vi "Process.vi"(8 "error in":errorcluster, 11 "Inst.Transport in":refnum<class "Inst.Transport.lvclass">) -> (0 "error out":errorcluster, 3 "Inst.Transport out":refnum<class "Inst.Transport.lvclass">)   [LabVIEW 2019, in "Inst.Transport.lvclass"]
doc: "---------------------------------------------------------------\nJKI State Machine Objects™\nhttp://jki.net/state-machine-objects/\nCopyright (C) 2005-2015, JKI <info@jki.net>\nALL RIGHTS RESERVED"
uses:
  Inst.Transport.lvclass
  C:/Program Files (x86)/National Instruments/LabVIEW 2019/vi.lib/JKI/JKI SMO/SMO/SMO.lvclass
  C:/Program Files (x86)/National Instruments/LabVIEW 2019/user.lib/LevyLab/Instrument Framework/Instrument/Instrument.lvclass
  Typedefs/Inst.Transport.PublicCommands--Enum.ctl
  Typedefs/Inst.Transport.ProtectedCommands--Enum.ctl
  Typedefs/startTransport--Request--Cluster.ctl
  Typedefs/Inst.Transport.Methods--Enum.ctl
  Typedefs/setExptFolder--Request--Cluster.ctl
  Typedefs/setExptComments--Request--Cluster.ctl
  Typedefs/PrivateEvents--MessageToProcess.ctl
  <userlib>/LevyLab/RemoteControl/RemoteControl/Typedefs/Message--Cluster.ctl
  Inst.Transport.lvclass/Inst.Transport.ctl
  Transport/Transport.lvclass/Transport.ctl
  Typedefs/Inst.Transport.Status--Enum.ctl
  <vilib>/JKI/JKI SMO/SMO/SMO.lvclass/SMO.ctl
  Control Experiment/Control Experiment.lvclass
  Control Experiment/Control Experiment.lvclass/Control Experiment.ctl
  Transport/Typedefs/Lockin_Sweep JSON--Cluster.ctl
  <userlib>/LevyLab/Lockin-Multichannel/Instrument.DAQ/Typedefs/Sweep.Channel--Cluster--Array.ctl
  <userlib>/LevyLab/Lockin-Multichannel/Instrument.DAQ/Typedefs/Sweep.Channel--Cluster.ctl
  <userlib>/LevyLab/Lockin-Multichannel/Instrument.DAQ/Typedefs/Sweep.Pattern--Enum.ctl
  Typedefs/setSweepConfig--Request--Cluster.ctl
  41101f9e-a4cc-4be1-b6e3-cc7aeb9eb354.vi
  d30b621e-3614-4fe5-8996-767b375fe1bd.vi
  744a5e80-96fd-41c3-bea5-87d1f33fb3b4.vi
  079e2b50-2307-4fef-96c7-ae8985376933.vi
  0da1cde2-b360-4fd3-820f-4bad75bb71e2.vi
  853791a9-a17a-427f-8d0f-8733465fb5f1.vi
  744a5e80-96fd-41c3-bea5-87d1f33fb3b4.vi/ff32358f-5752-4f64-93da-f1ac2c9d74ec.vi
  744a5e80-96fd-41c3-bea5-87d1f33fb3b4.vi/9c9ac127-68ea-437e-b2ce-e5ac86e17640.vi
  079e2b50-2307-4fef-96c7-ae8985376933.vi/61d47894-c364-4f02-849c-bb7b5c709336.vi
  079e2b50-2307-4fef-96c7-ae8985376933.vi/f9306059-c150-44a7-be15-9e180968e338.vi
  0da1cde2-b360-4fd3-820f-4bad75bb71e2.vi/fdcd5adf-08a1-451f-a2c4-4cbf930fc1d1.vi
  0da1cde2-b360-4fd3-820f-4bad75bb71e2.vi/a9b2ee84-03f9-4d18-8962-6d8dc3837a88.vi
  <vilib>/JKI/JKI SMO/SMO/Private/ReftoDVR--SMO.vi
  853791a9-a17a-427f-8d0f-8733465fb5f1.vi/4b7fe6b5-57cf-4521-ae99-b4f82cdb538d.vi
  853791a9-a17a-427f-8d0f-8733465fb5f1.vi/e7bc4215-eb92-4cc9-a4f3-d00d3197b518.vi
  <vilib>/Utility/Data Type/Get Type Information.vi
  <vilib>/Utility/Data Type/Get Numeric Information.vi
  <userlib>/_OpenG.lib/lvdata/lvdata.llb/Unwrap VVariant__ogtk.vi
  <vilib>/JDP Science/JSONtext/JSON text to Variant.vi
  <userlib>/LevyLab/Instrument Framework/Instrument/API/Instrument.sendMessageToProcess (variant).vi
  <vilib>/JDP Science/JSONtext/LVClass Serializer/JSONtext LVClass Serializer.lvclass
  <userlib>/LevyLab/Instrument Framework/Instrument Types/SCPI/Instrument.SCPI.lvclass
  <userlib>/LevyLab/Instrument Framework/Instrument/Instrument.lvclass
  <userlib>/LevyLab/RemoteControl/RemoteControl/RemoteControl.lvclass
  <userlib>/LevyLab/Debug/Debug.lvlib
  <vilib>/JKI/JKI SMO/SMO/SMO.lvclass
  Transport/Transport.lvclass
  <userlib>/LevyLab/Lockin-Multichannel/Instrument.DAQ/Instrument.DAQ.lvclass
  C:/Program Files (x86)/National Instruments/LabVIEW 2019/user.lib/LevyLab/Instrument Framework/Instrument Types/SCPI/Instrument.SCPI.lvclass
panel:
  in  "Tab Control":enum32{"Main", "Debug"}(tab)
  in  "stopTransport":bool
  out "Status":string
  in  "Close VI":bool
  in  "Open VI":bool
  in  "Ring":u16(ring)
  out "state history":string
  out "parameters":string
  out "command":string
  out "Secret Status":string
  # "Transport Server"
  # "Inst.Transport"
  # "For instructions on how to use the JKI State Machine Objects, examples and video tutorials, visit:\nhttp://jki.net/state-machine-objects/\n\nJKI State Machine Objects™\nhttp://jki.net/state-machine-objects/\nCopyright (C) 2005-2015, JKI <info@jki.net>\nALL RIGHTS RESERVED"
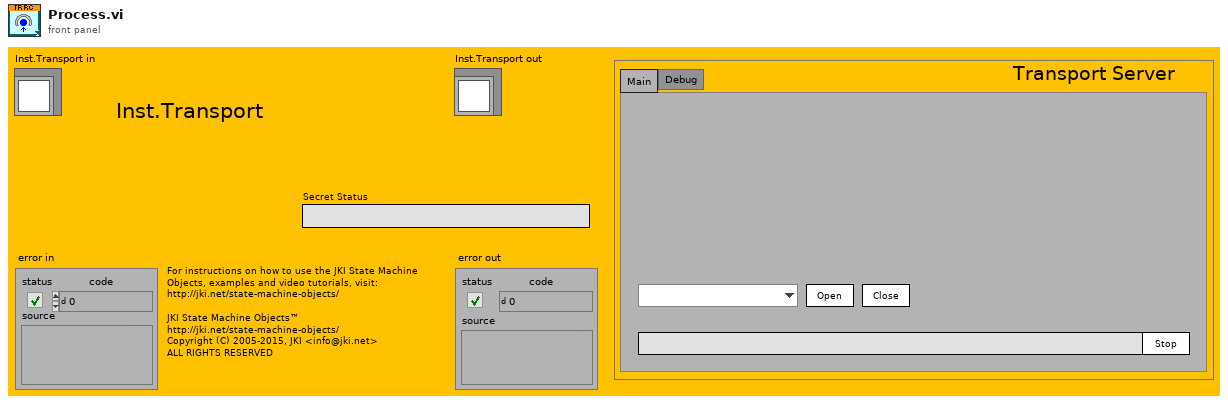
[diagram p1: front panel]
types:
  T1 = typedef "Inst.Transport.lvclass/Inst.Transport.ProtectedCommands--Enum.ctl" = enum16{"setStatus", "showUI", "hideUI"}
  T2 = typedef "Inst.Transport.lvclass/Inst.Transport.PublicCommands--Enum.ctl" = enum16{"startTransport", "stopTransport", "getStatus", "setExptFolder", "setExptComments", "appendExptParam", "clearExptParam", "setExptParam", "setSweepConfig"}
  T3 = typedef "Inst.Transport.lvclass/startTransport--Request--Cluster.ctl" = cluster{"method":T4}
  T4 = typedef "Inst.Transport.lvclass/Inst.Transport.Methods--Enum.ctl" = enum16{"LockinSweep", "LockinTime", "LockinTimeDelay"}
  T5 = typedef "Inst.Transport.lvclass/setExptFolder--Request--Cluster.ctl" = cluster{"folder":string}
  T6 = typedef "Inst.Transport.lvclass/setExptComments--Request--Cluster.ctl" = cluster{"comments":string}
  T7 = enum32{"invalid app kind", "Development System", "Run Time System", "Student Edition", "Embedded LabVIEW", "Evaluation", "Custom"}
  T8 = typedef "Inst.Transport.lvclass/Inst.Transport.Status--Enum.ctl" = enum16{"idle", "running"}
  T9 = enum32{"Invalid", "Standard", "Closed", "Hidden", "Minimized", "Maximized"}
  T10 = typedef "Inst.Transport.lvclass/setSweepConfig--Request--Cluster.ctl" = cluster{"sweepTime":dbl, "initialWaitTime":dbl, "returnToStart":bool, "sweepChannels":T11}
  T11 = typedef "Instrument.Lockin.lvlib/Instrument.DAQ.lvclass/Sweep.Channel--Cluster--Array.ctl" = T12[]
  T12 = typedef "Instrument.Lockin.lvlib/Instrument.DAQ.lvclass/Sweep.Channel--Cluster.ctl" = cluster{"Enable?":bool, "Channel":u16, "Start":dbl, "End":dbl, "Pattern":T13, "Table":dbl[]}
  T13 = typedef "Instrument.Lockin.lvlib/Instrument.DAQ.lvclass/Sweep.Pattern--Enum.ctl" = enum16{"Ramp /", "Ramp /\\", "Smooth Ramp _/", "Smooth Ramp _/\\_", "Table"}
  T14 = typedef "Transport.lvclass/Lockin_Sweep JSON--Cluster.ctl" = cluster{"Sweep Time (s)":dbl, "Initial Wait (s)":dbl, "Return to Start":bool, "Sweep Channels":T11, "Sweep Tables":cluster{"Ch":i32, "Table":dbl[]}[]}
  T15 = typedef "Inst.Transport.lvclass/PrivateEvents--MessageToProcess.ctl" = cluster{"Message":T16}
  T16 = typedef "RemoteControl.lvlib/RemoteControl.lvclass/Message--Cluster.ctl" = cluster{"Command":string, "Data":variant, "ID":string}
  T17 = cluster{"Core":cluster{"Current VI Reference":refnum<vi>, "Close Panel on Exit?":bool, "Last Error":cluster{"error":errorcluster, "previous state":string, "remaining states":string}, "Shutdown?":bool}, "SelfRef":refnum<class "Inst.Transport.lvclass">, "Transport":refnum<class "Transport.lvclass">, "C.E.":refnum<class "Control Experiment.lvclass">, "Folder":string, "Comments":string, "notifier":refnum<notifier>, "method":T4, "paths":path[], "path":path, "Running Step":i32, "sequence":string[], "MessageToProcess":T15, "UI Behavior":string, "wait":u32}
  T18 = cluster{"Current VI Reference":refnum<vi>, "Close Panel on Exit?":bool, "Last Error":cluster{"error":errorcluster, "previous state":string, "remaining states":string}, "Shutdown?":bool}
  T19 = typedef "Debug.lvlib/Attribute.Debug.lvclass/DebugBehavior.ctl" = enum16{"Normal", "Debug"}
  T20 = typedef "SMO.lvclass/Protected Events.ctl" = cluster{"StopProcesses":refnum<user-event>, "AbortProcesses":refnum<user-event>, "Config Changed":refnum<user-event>, "Dependency":refnum<user-event>}
  T21 = typedef "LV-Data.lvclass/Dictionary--cluster.ctl" = cluster{"key":string, "value":variant}
  T22 = typedef "Inst.Transport.lvclass/Inst.Transport.getAll--Cluster.ctl" = cluster{"data":variant}
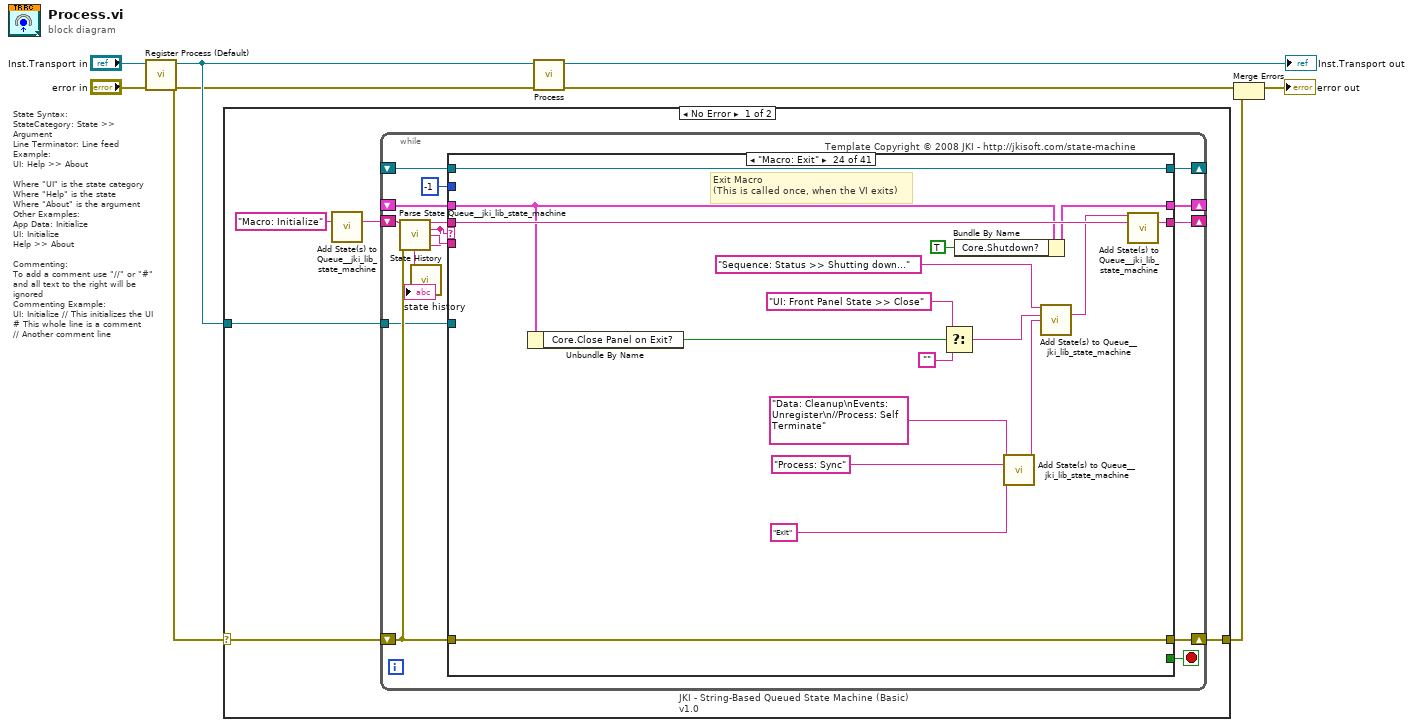
[diagram p0: block diagram]
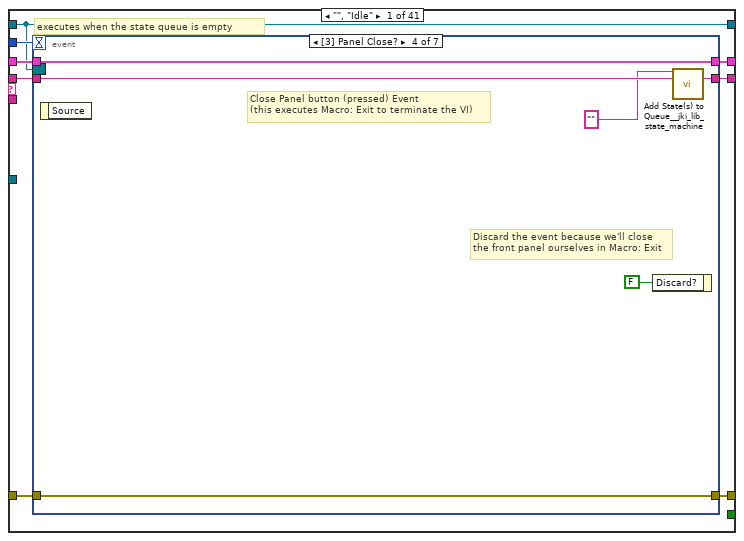
[diagram p2: hidden frame]
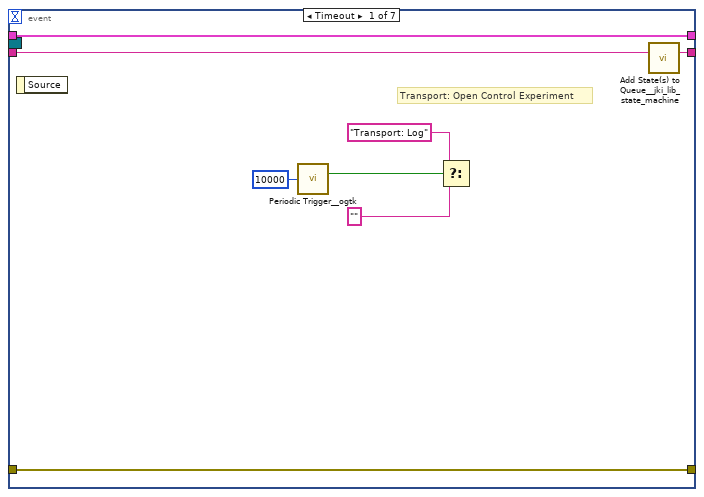
[diagram p3: hidden frame]
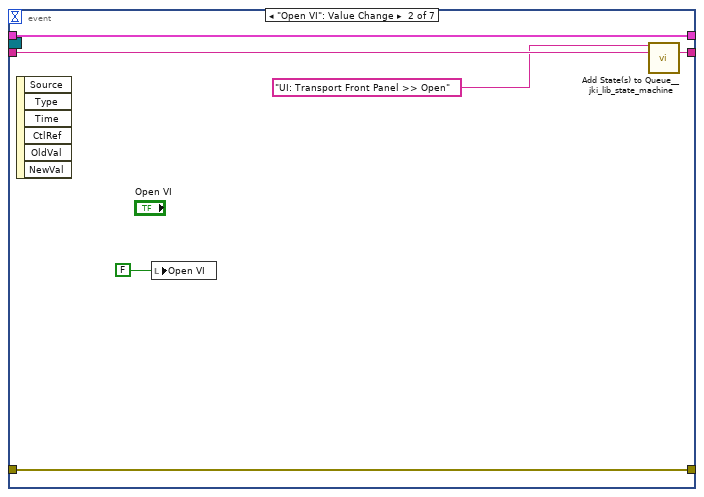
[diagram p4: hidden frame]
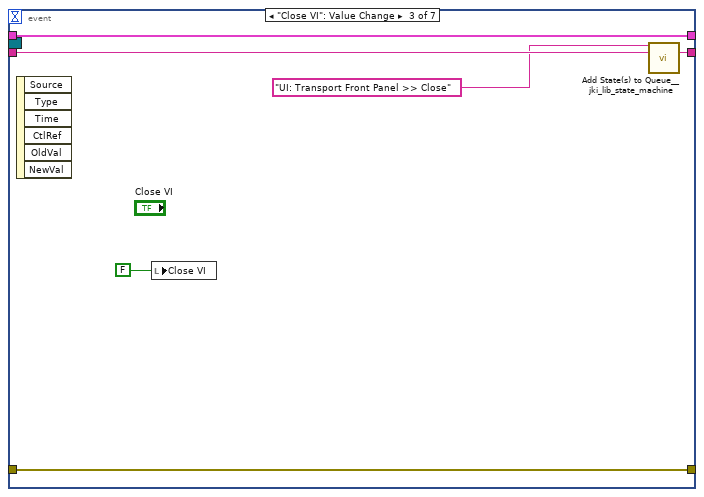
[diagram p5: hidden frame]
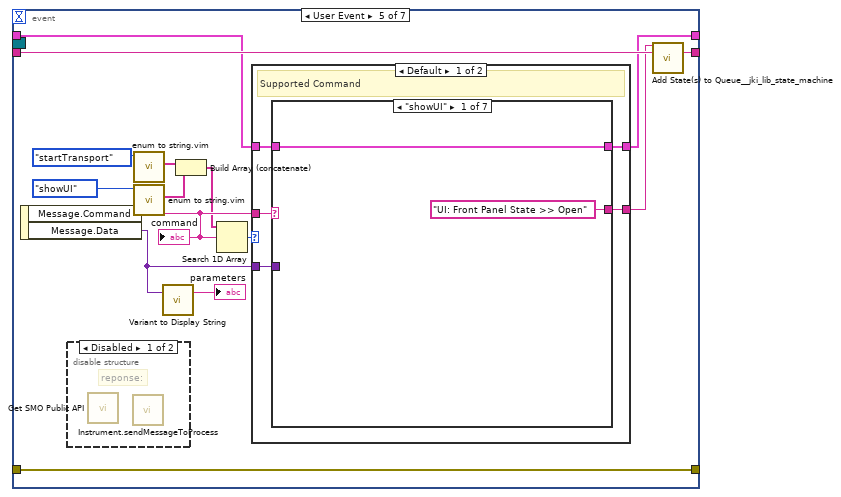
[diagram p6: hidden frame]
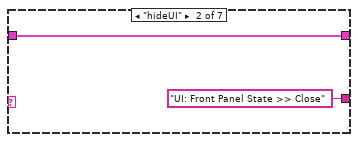
[diagram p8: hidden frame]
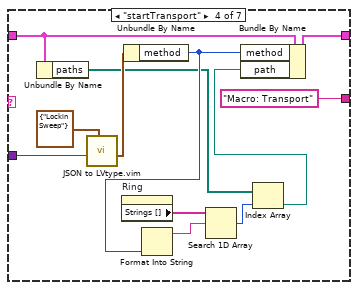
[diagram p10: hidden frame]
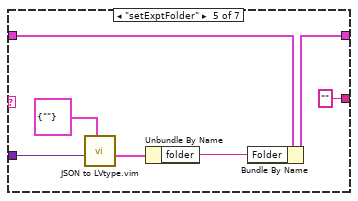
[diagram p11: hidden frame]
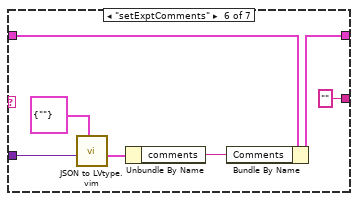
[diagram p12: hidden frame]
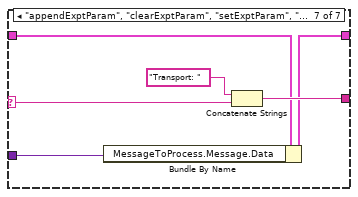
[diagram p13: hidden frame]
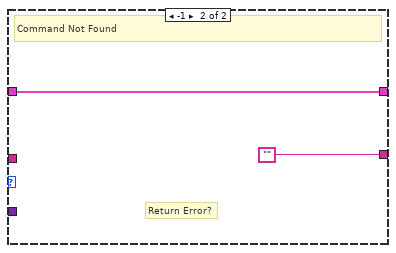
[diagram p14: hidden frame]
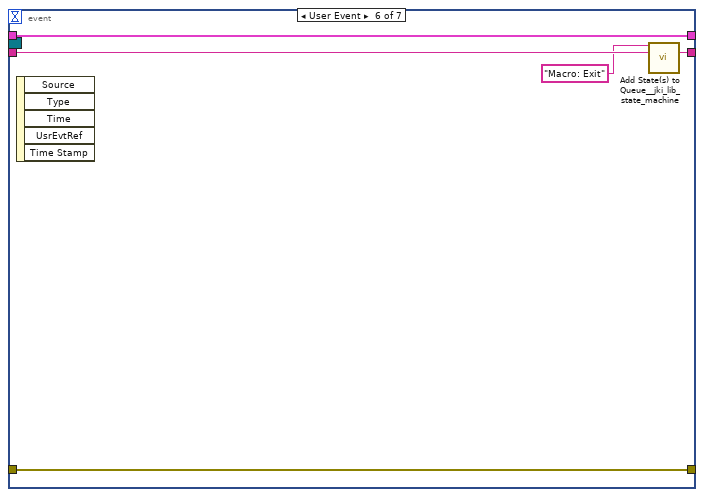
[diagram p15: hidden frame]
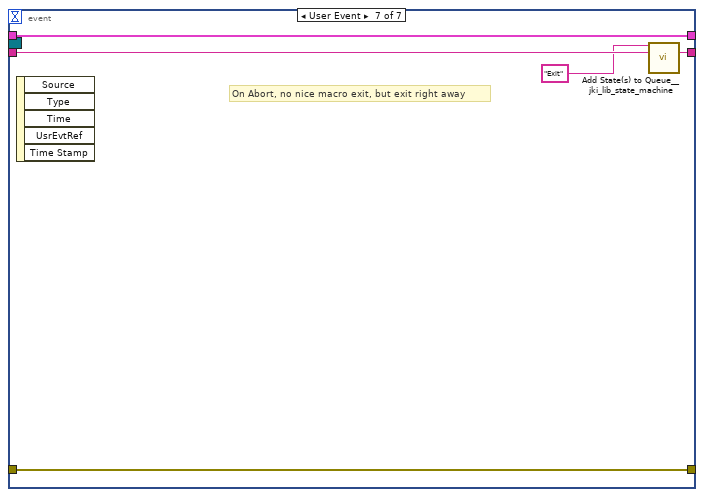
[diagram p16: hidden frame]
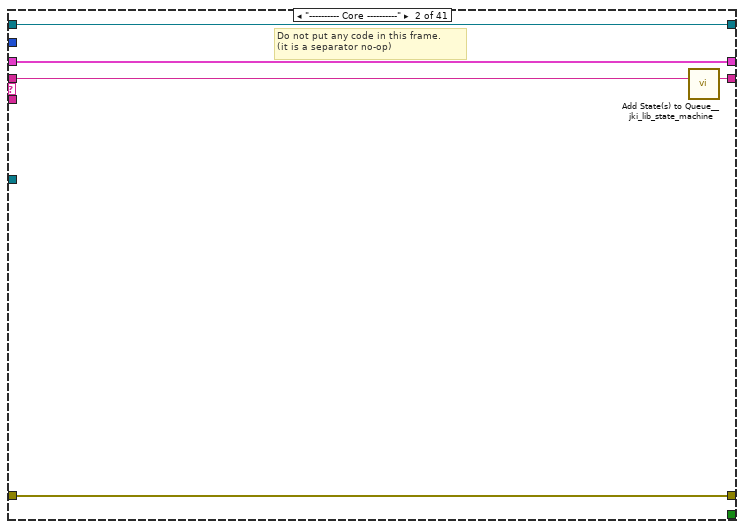
[diagram p17: hidden frame]
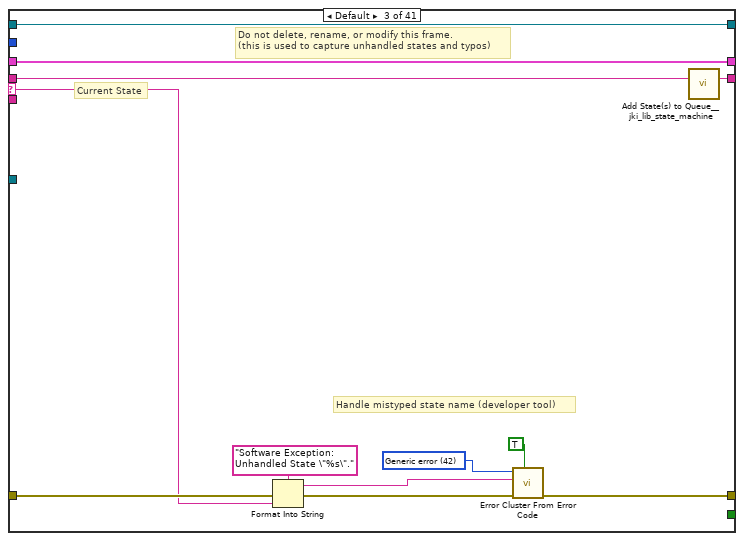
[diagram p18: hidden frame]
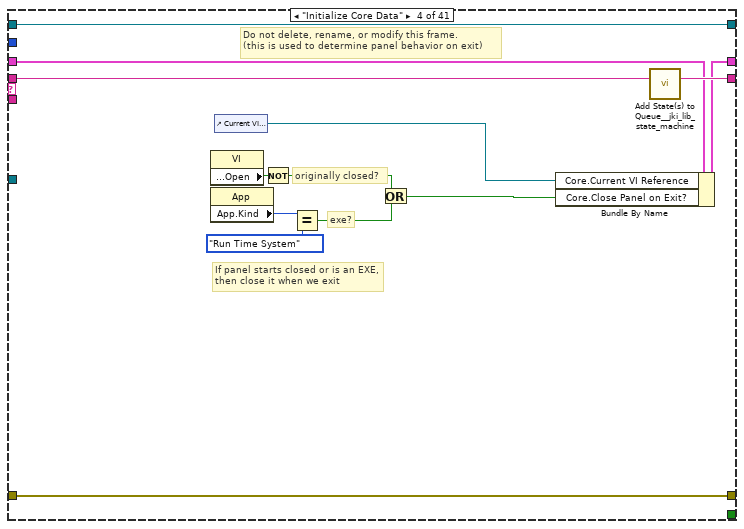
[diagram p19: hidden frame]
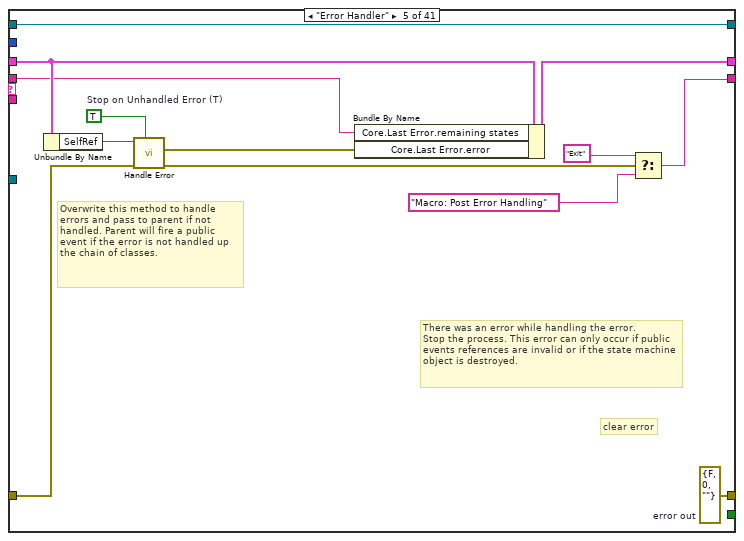
[diagram p20: hidden frame]
diagram:
  # "State Syntax:\nStateCategory: State >> Argument\nLine Terminator: Line feed\nExample:\nUI: Help >> About\n\nWhere \"UI\" is the state category\nWhere \"Help\" is the state\nWhere \"About\" is the argument\nOther Examples:\nApp Data: Initialize\nUI: Initialize\nHelp >> About\n\nCommenting:\nTo add a comment use \"//\" or \"#\" and all text to the right will be ignored\nCommenting Example:\nUI: Initialize // This initializes the UI\n# This whole line is a comment\n// Another comment line"
  n1 = call <vilib>:"Register Process (Default).vi"("error in (no error)"="error in", "SMO"="Inst.Transport in") -> ("error out"=w3:errorcluster, "SelfRef"=w6:refnum<class "Inst.Transport.lvclass">)  [unwired: 8 in]
  n2 = case shown="No Error" w3 {
    selector: w3 -> [w10 w687]
    tunnel: w6 -> [w11 _]
    tunnel: [w9 w687] -> w4
    frame No Error {
      n3 = call <vilib>:"Add State(s) to Queue__jki_lib_state_machine.vi"("State(s) in (\"\")"="Macro: Initialize") -> ("States Out"=w13:string)  [unwired: 14 in]
      n4 = while "JKI - String-Based Queued State Machine (Basic) v1.0" {
        shift-right: [w22] -> _
        shift-left: _ -> [w21]
        shift-right: [w25] -> w9
        shift-left: w10 -> [w19]
        shift-right: [w24] -> _
        shift-left: w13 -> [w26]
        tunnel: w11 -> [w18]
        shift-right: [w17] -> _
        shift-left: _ -> [w16]
        stop <- w23 stop-if-true
        # "Template Copyright © 2008 JKI - http://jkisoft.com/state-machine"
        n5 = call <vilib>:"Parse State Queue__jki_lib_state_machine.vi"("State Queue"=w26, "Error In (no error)"=w19) -> ("Remaining States"=w28:string, "Current State"=w15:string, "Arguments"=w27:string)  [unwired: 11 in]
        n6 = call <userlib>:"State History.vi"("Current State"=w15) -> ("History"=→"state history":string)  [unwired: 10 in]
        n7 = case shown="\"Macro: Exit\"" w15 {
          selector: w15 -> [_ _ w138 _ _ _ _ _ _ _ _ _ _ _ _ _ _ _ _ _ _ _ _ _ _ _ _ _ _ _ _ _ _ _ _ _ _ _ _ _ _]
          tunnel: w28 -> [w36 w136 w142 w161 w166 w180 w185 w206 w223 w246 w260 w265 w274 w283 w290 w306 w347 w380 w389 w401 w422 w437 w448 w465 w470 w481 w488 w493 w506 w512 w520 w544 w556 w604 w617 w624 w643 w656 w661 w667 w686]
          tunnel: w27 -> [_ _ _ _ _ _ _ _ _ w240 _ _ _ w275 w284 w300 w339 _ _ _ _ _ _ _ _ _ _ _ _ _ _ _ _ _ _ _ _ _ _ w662 w670]
          tunnel: w21 -> [w34 w133 w140 w152 w170 w176 w182 _ w218 w243 w255 w262 w272 w280 w288 w302 w338 w377 w386 w391 w412 w426 w445 w450 w467 w478 w485 w490 w499 w510 w515 w540 w553 w600 w613 w619 w639 w652 w657 w663 w676]
          tunnel: [w33 w134 w144 w158 w171 w175 w183 w197 w220 w236 w256 w263 w269 w281 w285 w303 w344 w378 w381 w399 w420 w425 w446 w453 w468 w472 w483 w491 w502 w508 w517 w528 w549 w597 w610 w621 w633 w650 w658 w664 w678] -> w25
          tunnel: w19 -> [w32 w134 w143 w158 w172 _ w183 w197 w220 w235 w257 w263 w268 w281 w286 w304 w343 w378 w381 w399 w420 w424 w446 w453 w468 w473 w482 w491 w496 w508 w517 w530 w548 w594 w608 w621 w634 w645 w658 w664 w672]
          tunnel: [w35 w135 w141 w160 w162 w179 w184 w205 w222 w245 w259 w264 w273 w282 w289 w305 w346 w379 w388 w400 w421 w436 w447 w464 w469 w480 w487 w492 w505 w511 w519 w543 w555 w603 w616 w623 w642 w655 w660 w666 w685] -> w24
          tunnel: [_ _ _ _ _ TRUE _ _ _ _ _ _ _ _ _ _ _ _ _ _ _ _ _ _ _ _ _ _ _ _ _ _ _ _ _ _ _ _ _ _ _] -> w23
          tunnel: [w31 w133 w140 w159 w169 w176 w182 w204 w219 w243 w255 w262 w272 w280 w288 w302 w338 w377 w386 w392 w413 w427 w445 w451 w467 w478 w485 w490 w499 w510 w516 w541 w553 w601 w614 w620 w640 w653 w657 w663 w675] -> w22
          tunnel: -1 ("Timeout") -> [w30 _ _ _ _ _ _ _ _ _ _ _ _ _ _ _ _ _ _ _ _ _ _ _ _ _ _ _ _ _ _ _ _ _ _ _ _ _ _ _ _]
          tunnel: w18 -> [_ _ _ _ _ _ _ w198 _ _ _ _ _ _ _ _ _ _ _ _ _ _ _ _ _ _ _ _ _ _ _ _ _ _ _ _ _ _ _ _ _]
          tunnel: [w29 w132 w137 w149 w174 w177 w181 w203 w221 w244 w254 w261 w271 w279 w287 w299 w345 w376 w387 w398 w419 w435 w444 w459 w466 w479 w486 w489 w504 w509 w518 w542 w554 w602 w615 w622 w641 w654 w659 w665 w684] -> w17
          tunnel: w16 -> [w29 w132 w137 w149 w174 w177 w181 w203 w221 w244 w254 w261 w271 w279 w287 w299 w345 w376 w387 w398 w419 w435 w444 w459 w466 w479 w486 w489 _ w509 w518 w542 w554 w602 w615 w622 w641 w654 w659 w665 w684]
          frame "", "Idle" {
            # "executes when the state queue is empty"
            n8 = event shown="[3] Panel Close?" {
              selector: w29 -> [_ _ _ _ _ _ _]
              dyn-events: _ -> [_ _ _ _ _ _ _]
              timeout: w30 -> [_ _ _ _ _ _ _]
              tunnel: w36 -> [w44 w50 w56 w62 w77 w126 w131]
              tunnel: [w43 w49 w55 w61 w76 w125 w130] -> w35
              tunnel: w34 -> [w41 w47 w53 w59 w71 w123 w128]
              tunnel: [w42 w48 w54 w60 w75 w124 w129] -> w33
              tunnel: w32 -> [w42 w48 w54 w60 w75 w124 w129]
              tunnel: [w41 w47 w53 w59 w70 w123 w128] -> w31
              event Timeout {
                # "Transport: Open Control Experiment"
                n9 = event-data() -> ()  [unwired: 1 in, 1 out]
                n10 = call <userlib>:"Periodic Trigger__ogtk.vi"("time (ms)"=u32 10000) -> ("Triggered"=w39:bool)  [unwired: 12 in, 2 out]
                n11 = Select(t="Transport: Log", s=w39, f="") -> ()  [unwired: 1 out]
                n12 = call <vilib>:"Add State(s) to Queue__jki_lib_state_machine.vi"("State(s) in (\"\")"=w44) -> ("States Out"=w43:string)  [unwired: 14 in]
              }
              event "Open VI": Value Change {
                n13 = event-data() -> ()  [unwired: 1 in, 6 out]
                n14 = local write "Open VI"(FALSE ("Open VI")) -> ()
                n15 = call <vilib>:"Add State(s) to Queue__jki_lib_state_machine.vi"("State(s) in Front (\"\")"="UI: Transport Front Panel >> Open" ("State(s) in Front (\"\")"), "State(s) in (\"\")"=w50) -> ("States Out"=w49:string)  [unwired: 13 in]
              }
              event "Close VI": Value Change {
                n16 = event-data() -> ()  [unwired: 1 in, 6 out]
                n17 = local write "Close VI"(FALSE ("Open VI")) -> ()
                n18 = call <vilib>:"Add State(s) to Queue__jki_lib_state_machine.vi"("State(s) in Front (\"\")"="UI: Transport Front Panel >> Close" ("State(s) in Front (\"\")"), "State(s) in (\"\")"=w56) -> ("States Out"=w55:string)  [unwired: 13 in]
              }
              event Panel Close? {
                # "Discard the event because we'll close the front panel ourselves in Macro: Exit"
                # "Close Panel button (pressed) Event\n(this executes Macro: Exit to terminate the VI)"
                n19 = event-data() -> ()  [unwired: 1 in, 1 out]
                n20 = event-data("Discard?"=FALSE) -> ()  [unwired: 1 in, 1 out]
                n21 = call <vilib>:"Add State(s) to Queue__jki_lib_state_machine.vi"("State(s) in Front (\"\")"="" ("f"), "State(s) in (\"\")"=w62) -> ("States Out"=w61:string)  [unwired: 13 in]
              }
              event User Event {
                n22 = event-data() -> ("Message.Command"=w69:string, "Message.Data"=w67:variant)  [unwired: 1 in]
                "command" <- w69
                n23 = disable-structure shown="Disabled" {
                  frame Disabled {
                    # "reponse:"
                    n24 = call-dynamic "Get SMO Public API.vi"() -> ()  [unwired: 9 in, 3 out]
                    n25 = call-poly <userlib>:"Instrument.sendMessageToProcess.vi"() -> ()  [unwired: 10 in, 2 out]
                  }
                  frame Enabled {
                  }
                }
                n26 = call "enum to string.vim"("enum in"=Inst.Transport.PublicCommands--Enum."startTransport" ("PublicCommands")) -> ("strings out"=w64:string[])  [unwired: 9 in, 1 out]
                n27 = call "enum to string.vim"("enum in"=Inst.Transport.ProtectedCommands--Enum."showUI" ("ProtectedCommands")) -> ("strings out"=w65:string[])  [unwired: 9 in, 1 out]
                n28 = call "Variant to Display String.vi"("Variant"=w67) -> ("xml string"=→"parameters":string)  [unwired: 2 in]
                n29 = Build Array (concatenate)(w64, w65) -> (w63:string[])
                n30 = Search 1D Array(1D array=w63, element=w69) -> (index of element=w74:i32)  [unwired: 1 in]
                n31 = case shown="Default" w74 {
                  tunnel: [w82 "" ("Empty String Constant")] -> w73
                  tunnel: w69 -> [w81 _]
                  tunnel: w67 -> [w80 _]
                  tunnel: w71 -> [w79 w120]
                  tunnel: [w78 w120] -> w70
                  frame Default {
                    # "Supported Command"
                    n32 = case shown="\"showUI\"" w81 {
                      selector: w81 -> [_ _ _ _ _ _ w118]
                      tunnel: ["UI: Front Panel State >> Open" ("State with Arguments") "UI: Front Panel State >> Close" ("State with Arguments") _ "Macro: Transport" "" ("State with Arguments") "" ("State with Arguments") w117] -> w82
                      tunnel: w80 -> [_ _ _ w96 w103 w110 w116]
                      tunnel: w79 -> [w84 w86 w87 w94 w106 w113 w114]
                      tunnel: [w84 w86 w87 w99 w105 w112 w115] -> w78
                      frame "showUI" {
                      }
                      frame "hideUI" {
                      }
                      frame Default {
                      }
                      frame "startTransport" {
                        n33 = Unbundle By Name(w94) -> ("paths"=w90:path[])
                        n34 = call "JSON to LVtype.vim"("type"=T3 {"method"=enum."LockinSweep"} ("startTransport"), "JSON Data in"=w96) -> ("Data out"=w97:T3)  [unwired: 8 in, 1 out]
                        n35 = property on="Ring" class="Ring (strict)"() -> ("Strings []"=w93:string[])  [unwired: 2 in, 2 out]
                        n36 = Unbundle By Name(w97) -> ("method"=w91:T4)
                        n37 = Format Into String(w91) -> (resulting string=w92:string)  [unwired: 3 in, 1 out]
                        n38 = Search 1D Array(1D array=w93, element=w92) -> (index of element=w89:i32)  [unwired: 1 in]
                        n39 = Index Array(array=w90, index=w89) -> (element=w88:path)
                        n40 = Bundle By Name(cluster=w94, "method"=w91, "path"=w88) -> (w99:T17)
                      }
                      frame "setExptFolder" {
                        n41 = call "JSON to LVtype.vim"("type"=T5 {"folder"=""} ("setExptFolder"), "JSON Data in"=w103) -> ("Data out"=w101:T5)  [unwired: 8 in, 1 out]
                        n42 = Unbundle By Name(w101) -> ("folder"=w100:string)
                        n43 = Bundle By Name(cluster=w106, "Folder"=w100) -> (w105:T17)
                      }
                      frame "setExptComments" {
                        n44 = call "JSON to LVtype.vim"("type"=T6 {"comments"=""} ("setExptComments"), "JSON Data in"=w110) -> ("Data out"=w108:T6)  [unwired: 8 in, 1 out]
                        n45 = Unbundle By Name(w108) -> ("comments"=w107:string)
                        n46 = Bundle By Name(cluster=w113, "Comments"=w107) -> (w112:T17)
                      }
                      frame "appendExptParam", "clearExptParam", "setExptParam", "setSweepConfig" {
                        n47 = Bundle By Name(cluster=w114, "MessageToProcess.Message.Data"=w116) -> (w115:T17)
                        n48 = Concatenate Strings("Transport: ", w118) -> (w117:string)
                      }
                    }
                  }
                  frame -1 {
                    # "Return Error?"
                    # "Command Not Found"
                  }
                }
                n49 = call <vilib>:"Add State(s) to Queue__jki_lib_state_machine.vi"("State(s) in Front (\"\")"=w73, "State(s) in (\"\")"=w77) -> ("States Out"=w76:string)  [unwired: 13 in]
              }
              event User Event {
                n50 = event-data() -> ()  [unwired: 1 in, 5 out]
                n51 = call <vilib>:"Add State(s) to Queue__jki_lib_state_machine.vi"("State(s) in Front (\"\")"="Macro: Exit", "State(s) in (\"\")"=w126) -> ("States Out"=w125:string)  [unwired: 13 in]
              }
              event User Event {
                # "On Abort, no nice macro exit, but exit right away"
                n52 = event-data() -> ()  [unwired: 1 in, 5 out]
                n53 = call <vilib>:"Add State(s) to Queue__jki_lib_state_machine.vi"("State(s) in Front (\"\")"="Exit", "State(s) in (\"\")"=w131) -> ("States Out"=w130:string)  [unwired: 13 in]
              }
            }
          }
          frame "---------- Core ----------" {
            # "Do not put any code in this frame.\n(it is a separator no-op)"
            n54 = call <vilib>:"Add State(s) to Queue__jki_lib_state_machine.vi"("State(s) in (\"\")"=w136) -> ("States Out"=w135:string)  [unwired: 14 in]
          }
          frame Default {
            w147 = 42 items=["No error", "Argument error", "Memory is full", "Out of zone", "End of file", "File already open", "Generic file I/O error", "File not found", "File permission error", "Disk is full", "Duplicate path", "Too many files open", "System feature not enabled", "Resource file not found", "Cannot add resource", "Resource not found", "Image not found", "Image memory error", "Pen does not exist", "Config type invalid", "Config token not found", "Config parse error", "Config memory error", "Bad external code format", "Bad external code offset", "External code not present", "Null window", "Destroy window error", "Null menu", "Print aborted", "Bad print record", "Print driver error", "Windows error during printing", "Memory error during printing", "Print dialog error", "Generic print error", "Invalid device refnum", "Device not found", "Device parameter error", "Device unit error", "Cannot open device", "Device call aborted", "Generic error", "Cancelled by user", "Object ID too low", "Object ID too high", "Object not in heap", "Unknown heap", "Unknown object (invalid DefProc)", "Unknown object (DefProc not in table)", "Message out of range", "Invalid (null) method", "Unknown message", "Manager call not supported", "Bad address", "Network operation in progress", "Network operation timed out", "Connection is busy", "Network attribute not supported", "Network error", "Address in use", "System out of memory", "Connection aborted", "Connection refused", "Not connected", "Already connected", "Connection closed", "Initialization error (interapplication manager)", "Bad occurrence", "Wait on unbound occurrence handler", "Occurrence queue overflow", "Datalog type conflict", "Unused", "Unrecognized type (interapplication manager)", "Memory corrupt", "Failed to make temporary DLL", "Old CIN version", "Drag socket not found", "Failed to load drop-object", "Failed to register OLE object", "Failed to release OLE object", "Format specifier type mismatch", "Unknown format specifier", "Too few format specifiers", "Too many format specifiers", "Scan failed", "Newer CIN version", "Error converting to variant", "Runtime menu error", "Password tampered", "Variant attribute not found", "Incompatible variant data type", "Event data is not available", "Event Store is not present", "Occurrence is not found", "Event Queue is not created", "Event info is not available", "Refnum passed is NULL", "Error retrieving Class GUID", "Error retrieving CoClass GUID", "Error retrieving TypeLib GUID.", "Bad built application magic bytes.", "Specific driver is different from the specific driver associated with the Logical Name.", "There is no session opened to the class driver.", "Max Error", "MAX - Error with config objects", "MAX - Error loading configuration", "MAX - Group not supported"]
            # "Current State"
            # "Do not delete, rename, or modify this frame.\n(this is used to capture unhandled states and typos)"
            # "Handle mistyped state name (developer tool)"
            n55 = Format Into String(format string="Software Exception: Unhandled State \"%s\"." ("message"), error in=w143, w138) -> (resulting string=w146:string, error out=w145:errorcluster)  [unwired: 1 in]
            n56 = call <vilib>:"Error Cluster From Error Code.vi"("show call chain? (False)"=TRUE, "error in (no error)"=w145, "error message (\"\")"=w146, "error code (0)"=w147) -> ("error out"=w144:errorcluster)  [unwired: 5 in]
            n57 = call <vilib>:"Add State(s) to Queue__jki_lib_state_machine.vi"("State(s) in (\"\")"=w142) -> ("States Out"=w141:string)  [unwired: 14 in]
          }
          frame "Initialize Core Data" {
            # "Do not delete, rename, or modify this frame.\n(this is used to determine panel behavior on exit)"
            # "originally closed?"
            # "exe?"
            # "If panel starts closed or is an EXE, then close it when we exit"
            n58 = property class="VI"() -> ("Front Panel.Open"=w157:bool)  [unwired: 2 in, 2 out]
            n59 = property class="App"() -> ("App.Kind"=w156:T7)  [unwired: 2 in, 2 out]
            n60 = control-ref of="Current VI Reference"() -> (w150:refnum<vi>)
            n61 = Not(x=w157) -> (.not. x?=w154:bool)
            n62 = Equal?(x=w156, y=T7."Run Time System" ("Application:Kind")) -> (x = y?=w153:bool)
            n63 = Or(x=w154, y=w153) -> (x .or. y?=w151:bool)
            n64 = Bundle By Name(cluster=w152, "Core.Current VI Reference"=w150, "Core.Close Panel on Exit?"=w151) -> (w159:T17)
            n65 = call <vilib>:"Add State(s) to Queue__jki_lib_state_machine.vi"("State(s) in (\"\")"=w161) -> ("States Out"=w160:string)  [unwired: 14 in]
          }
          frame "Error Handler" {
            w167 = TRUE  # Stop on Unhandled Error (T)
            w171 = errorcluster {"status"=FALSE, "code"=0, "source"=""}  # error out
            # "clear error"
            # "There was an error while handling the error.\nStop the process. This error can only occur if public events references are invalid or if the state machine object is destroyed."
            # "Overwrite this method to handle errors and pass to parent if not handled. Parent will fire a public event if the error is not handled up the chain of classes."
            n66 = Unbundle By Name(w170) -> ("SelfRef"=w173:refnum<class "Inst.Transport.lvclass">)
            n67 = call-dynamic "Handle Error.vi"("Stop on Unhandled Error (T)"=w167, "error in"=w172, "SMO"=w173) -> ("handling error"=w163:errorcluster, "Unhandled error"=w168:errorcluster)  [unwired: 6 in, 1 out]
            n68 = Bundle By Name(cluster=w170, "Core.Last Error.remaining states"=w166, "Core.Last Error.error"=w168) -> (w169:T17)
            n69 = Select(t="Exit", s=w163, f="Macro: Post Error Handling") -> (s? t:f=w162:string)
          }
          frame "Exit" {
            # "Do not put any code in this frame.\n(No errors that occur here will be handled.)"
            n70 = Unbundle By Name(w176) -> ("Core.Last Error.error"=w175:errorcluster)
            n71 = call <vilib>:"Add State(s) to Queue__jki_lib_state_machine.vi"("State(s) in (\"\")"=w180) -> ("States Out"=w179:string)  [unwired: 14 in]
          }
          frame "---------- Data ----------" {
            # "Do not put any code in this frame.\n(It is a separator no-op. You can make a copy of this frame to create a new Data frame)"
            n72 = call <vilib>:"Add State(s) to Queue__jki_lib_state_machine.vi"("State(s) in (\"\")"=w185) -> ("States Out"=w184:string)  [unwired: 14 in]
          }
          frame "Data: Initialize" {
            w186 = path ""  # path
            w187 = path[] []  # paths
            w188 = Inst.Transport.Methods--Enum."LockinSweep"  # method
            w195 = u32 0  # wait
            w196 = ""  # UI Behavior
            w199 = T15 {"Message"={"Command"="", "Data"=variant(string ""), "ID"=""}}  # MessageToProcess
            w200 = string[] []  # sequence
            w201 = -1  # Running Step
            w202 = T18 {"Current VI Reference"=refnum, "Close Panel on Exit?"=FALSE, "Last Error"={"error"={"status"=FALSE, "code"=0, "source"=""}, "previous state"="", "remaining states"=""}, "Shutdown?"=FALSE}  # Core
            # "do not delete - used by framework"
            # "Initialize the shift-register data, here.\n(data names are defined by what you wire into the bundle function)"
            n73 = Unbundle By Name(w198) -> ("Transport"=w189:refnum<class "Transport.lvclass">, "Folder"=w191:string, "Comments"=w190:string, "notifier"=w194:refnum<notifier>)
            n74 = call "Read Dependencies.vi"("Transport"=w189) -> ("C.E."=w192:refnum<class "Control Experiment.lvclass">, "Transport"=w193:refnum<class "Transport.lvclass">)  [unwired: 8 in, 1 out]
            n75 = Bundle("Core"=w202, "SelfRef"=w198, "Transport"=w193, "C.E."=w192, "Folder"=w191, "Comments"=w190, "notifier"=w194, "method"=w188, "paths"=w187, "path"=w186, "Running Step"=w201, "sequence"=w200, "MessageToProcess"=w199, "UI Behavior"=w196, "wait"=w195) -> (w204:T17)  [unwired: 1 in]
            n76 = call <vilib>:"Add State(s) to Queue__jki_lib_state_machine.vi"("State(s) in (\"\")"=w206) -> ("States Out"=w205:string)  [unwired: 14 in]
          }
          frame "Data: Populate Ring" {
            n77 = call <userlib>:"User Library__ogtk.vi"() -> ("User Library (+ Relative)"=w207:path)  [unwired: 1 in]
            n78 = Unbundle By Name(w218) -> ("SelfRef"=w216:refnum<class "Inst.Transport.lvclass">, "Transport"=w217:refnum<class "Transport.lvclass">)
            n79 = call <vilib>:"Delimited String to 1D String Array.vi"("delimiter"="\n" ("delimiter (Tab)"), "delimited string"="Lockin_time.vi\nLockin_sweep.vi\nTHz_TimeDelay.vi") -> ("string array"=w212:string[])  [unwired: 9 in]
            n80 = call <vilib>:"Delimited String to 1D String Array.vi"("delimiter"="\n" ("delimiter (Tab)"), "delimited string"="LockinTime\nLockinSweep\nLockinTimeDelay") -> ("string array"=w209:string[])  [unwired: 9 in]
            n81 = for {
              tunnel: [w224] -> w213 mode=indexing if=w226
              tunnel: [w230] -> w214 mode=indexing if=w226
              tunnel: w209 -> [w230] mode=indexing
              tunnel: w212 -> [w229] mode=indexing
              tunnel: w207 -> [w228]
              n82 = call <vilib>:"Recursive File List.vi"("pattern"=w229, "Folder Path"=w228) -> ("All Files in Dir"=w227:path[])  [unwired: 5 in, 4 out]
              n83 = Index Array(array=w227) -> (element=w225:path)  [unwired: 1 in]
              n84 = call <vilib>:"Check if File or Folder Exists.vi"("path"=w225) -> ("file or folder exists?"=w226:bool, "dup path"=w224:path)  [unwired: 8 in, 1 out]
            }
            n85 = Bundle By Name(cluster=w218, "SelfRef"=w216, "Transport"=w217, "paths"=w213) -> (w219:T17)
            n86 = property on="Ring" class="Ring (strict)"("Strings []"=w214) -> ()  [unwired: 2 in, 2 out]
            n87 = call <vilib>:"Add State(s) to Queue__jki_lib_state_machine.vi"("State(s) in (\"\")"=w223) -> ("States Out"=w222:string)  [unwired: 14 in]
          }
          frame "Data: Set Status" {
            # "Dat: Set Status.\n()"
            n88 = Unbundle By Name(w243) -> ("SelfRef"=w238:refnum<class "Inst.Transport.lvclass">, "method"=w242:T4)
            n89 = Scan From String(input string=w240, default 1=Inst.Transport.Status--Enum."running" ("Status")) -> (output 1=w237:T8)  [unwired: 3 in, 3 out]
            n90 = case shown="\"running\"" w237 {
              selector: w237 -> [_ w250]
              tunnel: ["" w253] -> w232
              tunnel: w242 -> [_ w251]
              tunnel: [FALSE ("Visible") TRUE ("Visible")] -> w231
              frame "idle", Default {
              }
              frame "running" {
                n91 = Format Into String(format string="%s: %s", w251, w250) -> (resulting string=w253:string)  [unwired: 2 in, 1 out]
              }
            }
            n92 = property on="stopTransport" class="Bool (strict)"("Visible"=w231) -> ()  [unwired: 2 in, 2 out]
            n93 = call <vilib>:"Build State String with Arguments__JKI_lib_State_Machine.vi"("Arguments (\"\")"=w232, "State"="Sequence: Status") -> ("State with Arguments"=w234:string)  [unwired: 4 in]
            n94 = call-poly <userlib>:"Instrument.sendMessageToProcess.vi"("error in (no error)"=w235, "Data"=w237, "Command"=Inst.Transport.ProtectedCommands--Enum."setStatus" ("ProtectedCommands"), "Instrument"=w238) -> ("error out"=w236:errorcluster)  [unwired: 6 in, 1 out]
            n95 = call <vilib>:"Add State(s) to Queue__jki_lib_state_machine.vi"("State(s) in Front (\"\")"=w234, "State(s) in (\"\")"=w246) -> ("States Out"=w245:string)  [unwired: 13 in]
          }
          frame "Data: Cleanup" {
            # "Cleanup any data and references, here.\n(this is called automatically, by the Macro: Exit)"
            n96 = Unbundle By Name(w255) -> ("Core.Current VI Reference"=w258:refnum<vi>)
            n97 = Close Reference(reference=w258, error in (no error)=w257) -> (error out=w256:errorcluster)
            n98 = call <vilib>:"Add State(s) to Queue__jki_lib_state_machine.vi"("State(s) in (\"\")"=w260) -> ("States Out"=w259:string)  [unwired: 14 in]
          }
          frame "---------- UI ----------" {
            # "Do not put any code in this frame.\n(It is a separator no-op. You can make a copy of this frame to create a new UI frame)"
            n99 = call <vilib>:"Add State(s) to Queue__jki_lib_state_machine.vi"("State(s) in (\"\")"=w265) -> ("States Out"=w264:string)  [unwired: 14 in]
          }
          frame "UI: Initialize" {
            w266 = FALSE ("stopTransport")
            # "Initialize the User Interface, here.\n(this is called automatically, by the Macro: Init)"
            n100 = call <userlib>:"Fit VI window to Largest Dec__ogtk.vi"("error in (no error)"=w268, "border spacing (2 px)"=0) -> ("error out"=w269:errorcluster)  [unwired: 4 in, 1 out]
            n101 = local write "Open VI"(w266) -> ()
            n102 = local write "stopTransport"(w266) -> ()
            n103 = property on="stopTransport" class="Bool (strict)"("Visible"=w266) -> ()  [unwired: 2 in, 2 out]
            n104 = local write "Tab Control"(enum32{"Main", "Debug"}."Main" ("Tab Control")) -> ()
            n105 = call <vilib>:"Add State(s) to Queue__jki_lib_state_machine.vi"("State(s) in (\"\")"=w274) -> ("States Out"=w273:string)  [unwired: 14 in]
          }
          frame "UI: Wait" {
            # "Do not put any code in this frame.\n(It is a separator no-op. You can make a copy of this frame to create a new UI frame)"
            n106 = Scan From String(format string="%d", input string=w275, default 1=u32 0 ("default value 1")) -> (output 1=w276:u32)  [unwired: 2 in, 3 out]
            n107 = Wait (ms)(milliseconds to wait=w276) -> ()  [unwired: 1 out]
            n108 = call <vilib>:"Add State(s) to Queue__jki_lib_state_machine.vi"("State(s) in (\"\")"=w283) -> ("States Out"=w282:string)  [unwired: 14 in]
          }
          frame "UI: Cursor Set" {
            # "Argument"
            # "Initialize the User Interface, here.\n(this is called automatically, by the Macro: Init)"
            n109 = disable-structure shown="Default" {
              disable-tunnel: w286 -> [w291 w294]
              disable-tunnel: [w291 w293] -> w285
              disable-tunnel: w284 -> [_ w292]
              frame condition #0 {
              }
              frame condition #1 (active) {
                n110 = case shown="\"Idle\", Default" w292 {
                  tunnel: w294 -> [w296 w298]
                  tunnel: [w295 w297] -> w293
                  frame "Idle", Default {
                    n111 = call <vilib>:"Unset Busy.vi"("error in (no error)"=w296) -> ("error out"=w295:errorcluster)  [unwired: 10 in]
                  }
                  frame "Busy" {
                    n112 = call <vilib>:"Set Busy.vi"("error in (no error)"=w298) -> ("error out"=w297:errorcluster)  [unwired: 9 in, 1 out]
                  }
                }
              }
            }
            n113 = call <vilib>:"Add State(s) to Queue__jki_lib_state_machine.vi"("State(s) in (\"\")"=w290) -> ("States Out"=w289:string)  [unwired: 14 in]
          }
          frame "UI: Front Panel State" {
            # "Argument"
            # "Set Front Panel Open or Closed\n(Usage: \"UI: Front Panel State >> Open|Close\")"
            n114 = Unbundle By Name(w302) -> ("Core.Current VI Reference"=w301:refnum<vi>)
            n115 = disable-structure shown="Default" {
              disable-tunnel: w304 -> [w310 w333]
              disable-tunnel: [w309 w333] -> w303
              disable-tunnel: w301 -> [w308 _]
              disable-tunnel: w300 -> [w307 _]
              frame condition #0 (active) {
                n116 = case shown="\"Open\", Default" w307 {
                  tunnel: w310 -> [w314 w327]
                  tunnel: [w316 w328] -> w309
                  tunnel: w308 -> [w315 w325]
                  frame "Open", Default {
                    n117 = property class="VI"(reference=w315, error in=w314) -> (reference out=w312:refnum<vi>, error out=w313:errorcluster, "FP.State"=w311:T9)
                    n118 = case shown="\"Closed\"" w311 {
                      tunnel: [w319 w322] -> w316
                      tunnel: w313 -> [w318 w322]
                      tunnel: w312 -> [w317 _]
                      frame "Closed" {
                        n119 = invoke class="VI" method="FP.Open"(reference=w317, error in=w318, "Activate"=TRUE, "State"=T9."Standard") -> (error out=w319:errorcluster)  [unwired: 1 in, 4 out]
                      }
                      frame Default {
                      }
                    }
                  }
                  frame "Close" {
                    n120 = property class="VI"(reference=w325, error in=w327) -> (reference out=w324:refnum<vi>, error out=w326:errorcluster, "FP.State"=w323:T9)
                    n121 = case shown="Default" w323 {
                      tunnel: [w329 w332] -> w328
                      tunnel: w326 -> [w329 w331]
                      tunnel: w324 -> [_ w330]
                      frame "Invalid", "Closed" {
                      }
                      frame Default {
                        n122 = invoke class="VI" method="FP.Close"(reference=w330, error in=w331) -> (error out=w332:errorcluster)  [unwired: 1 in, 2 out]
                      }
                    }
                  }
                }
              }
              frame condition #1 {
              }
            }
            n123 = call <vilib>:"Add State(s) to Queue__jki_lib_state_machine.vi"("State(s) in (\"\")"=w306) -> ("States Out"=w305:string)  [unwired: 14 in]
          }
          frame "UI: Transport Front Panel" {
            n124 = Unbundle By Name(w338) -> ("paths"=w341:path[])
            n125 = Index Array(array=w341, index="Ring") -> (element=w342:path)
            n126 = Open VI Reference(vi path=w342, error in (no error)=w343) -> (vi reference=w336:refnum<vi>, error out=w337:errorcluster)  [unwired: 4 in]
            n127 = case shown="\"Open\", Default" w339 {
              tunnel: w337 -> [w352 w368]
              tunnel: [w354 w369] -> w334
              tunnel: w336 -> [w353 w366]
              tunnel: [w348 w363] -> w335
              frame "Open", Default {
                n128 = property class="VI"(reference=w353, error in=w352) -> (reference out=w350:refnum<vi>, error out=w351:errorcluster, "FP.State"=w349:T9)
                n129 = case shown="Default" w349 {
                  tunnel: [w358 w362] -> w354
                  tunnel: w351 -> [w357 w362]
                  tunnel: w350 -> [w356 w361]
                  tunnel: [w355 w361] -> w348
                  frame Default {
                    n130 = invoke class="VI" method="FP.Open"(reference=w356, error in=w357, "Activate"=TRUE, "State"=T9."Standard") -> (reference out=w355:refnum<vi>, error out=w358:errorcluster)  [unwired: 1 in, 3 out]
                  }
                  frame "Invalid" {
                  }
                }
              }
              frame "Close" {
                n131 = property class="VI"(reference=w366, error in=w368) -> (reference out=w365:refnum<vi>, error out=w367:errorcluster, "FP.State"=w364:T9)
                n132 = case shown="Default" w364 {
                  tunnel: [w371 w375] -> w369
                  tunnel: w367 -> [w371 w374]
                  tunnel: w365 -> [w370 w373]
                  tunnel: [w370 w372] -> w363
                  frame "Invalid", "Closed" {
                  }
                  frame Default {
                    n133 = invoke class="VI" method="FP.Close"(reference=w373, error in=w374) -> (reference out=w372:refnum<vi>, error out=w375:errorcluster)  [unwired: 1 in, 1 out]
                  }
                }
              }
            }
            n134 = Close Reference(reference=w335, error in (no error)=w334) -> (error out=w344:errorcluster)
            n135 = call <vilib>:"Add State(s) to Queue__jki_lib_state_machine.vi"("State(s) in (\"\")"=w347) -> ("States Out"=w346:string)  [unwired: 14 in]
          }
          frame "---------- Macro ----------" {
            # "Do not put any code in this frame.\n(It is a separator no-op. You can make a copy of this frame to create a new Macro frame)"
            n136 = call <vilib>:"Add State(s) to Queue__jki_lib_state_machine.vi"("State(s) in (\"\")"=w380) -> ("States Out"=w379:string)  [unwired: 14 in]
          }
          frame "Macro: Initialize" {
            # "Initialization Macro\n(This is called once, when the VI starts)"
            n137 = call <vilib>:"Add State(s) to Queue__jki_lib_state_machine.vi"("State(s) in Front (\"\")"="Data: Initialize\nInitialize Core Data\nEvents: Register", "State(s) in (\"\")"="Process: Sync", "State(s) at Back (\"\")"="UI: Initialize\nUI: Front Panel State >> Close\nSequence: Status >> Initializing...\nMacro: Debug\nData: Populate Ring\nSequence: Status") -> ("States Out"=w384:string)  [unwired: 12 in]
            n138 = call <vilib>:"Add State(s) to Queue__jki_lib_state_machine.vi"("State(s) in Front (\"\")"=w384, "State(s) in (\"\")"=w389) -> ("States Out"=w388:string)  [unwired: 13 in]
          }
          frame "Macro: Post Error Handling" {
            # "Clear Last Error?"
            n139 = Unbundle By Name(w391) -> ("Core.Last Error.remaining states"=w393:string, "Core.Shutdown?"=w394:bool)
            n140 = Unbundle By Name(w391) -> ("Core.Last Error.error"=w397:errorcluster)
            n141 = case shown="False" FALSE {
              tunnel: w397 -> [w405 _]
              tunnel: [w405 _] -> w396
              frame False {
              }
              frame True {
              }
            }
            n142 = case shown="False" w394 {
              tunnel: w393 -> [w402 w404]
              tunnel: [w402 w403] -> w390
              frame False {
                # "These are the remaining states (at the moment the error occured). States can be altered according to business logic."
                # "NOT SHUTTING DOWN"
              }
              frame True {
                # "Developer can decide to alter the states but should be aware that during the shutdown process, there are certain states that must be run for the SMO to properly shut itself (and this process) down. As such, one can add states to perform additional clean-ups, but should append the remaining state to be executed."
                # "SHUTTING DOWN"
                n143 = call <vilib>:"Add State(s) to Queue__jki_lib_state_machine.vi"("State(s) in (\"\")"=w404) -> ("States Out"=w403:string)  [unwired: 14 in]
              }
            }
            n144 = Bundle By Name(cluster=w391, "Core.Last Error.error"=w396) -> (w392:T17)
            n145 = call <vilib>:"Add State(s) to Queue__jki_lib_state_machine.vi"("State(s) in Front (\"\")"=w390, "State(s) in (\"\")"=w401) -> ("States Out"=w400:string)  [unwired: 13 in]
          }
          frame "Macro: Run Sequence" {
            # "0,1,2,3,4,"
            # "5"
            # "Do not put any code in this frame.\n(It is a separator no-op. You can make a copy of this frame to create a new Macro frame)"
            n146 = Unbundle By Name(w412) -> ("sequence"=w408:string[], "Running Step"=w406:i32)
            n147 = Array Size(array=w408) -> (size(s)=w418:i32)
            n148 = Index Array(array=w408, index=w406) -> (element=w407:string)
            n149 = Greater Or Equal?(x=w418, y=w406) -> (x >= y?=w410:bool)
            n150 = Select(t=-1 ("Running Step"), s=w410, f=w406) -> (s? t:f=w417:i32)
            n151 = Bundle By Name(cluster=w412, "Running Step"=w417) -> (w413:T17)
            n152 = Select(t="Sequence: Status >> ...", s=w410, f="Idle //Check Event Structure\nMacro: Run Sequence" ("State(s) at Back (\"\")")) -> (s? t:f=w409:string)
            n153 = call <vilib>:"Add State(s) to Queue__jki_lib_state_machine.vi"("State(s) in Front (\"\")"=w407, "State(s) at Back (\"\")"=w409) -> ("States Out"=w411:string)  [unwired: 13 in]
            n154 = call <vilib>:"Add State(s) to Queue__jki_lib_state_machine.vi"("State(s) in Front (\"\")"=w411, "State(s) in (\"\")"=w422) -> ("States Out"=w421:string)  [unwired: 13 in]
          }
          frame "Macro: Debug" {
            # "exe?"
            # "If pane is an EXE, then close it when we exit"
            # "Macro: Debug\n(get debug behavior, determine UI and determine shutdown behavior)"
            n155 = Unbundle By Name(w426) -> ("Core.Close Panel on Exit?"=w429:bool, "SelfRef"=w434:refnum<class "Inst.Transport.lvclass">)
            n156 = property class="App"() -> ("App.Kind"=w432:T7)  [unwired: 2 in, 2 out]
            n157 = Equal?(x=w432, y=T7."Run Time System" ("Application:Kind")) -> (x = y?=w428:bool)
            n158 = call <userlib>:"Get Debug Mode.vi"("error in (no error)"=w424, "SMO"=w434) -> ("error out"=w425:errorcluster, "Behavior"=w433:T19)  [unwired: 7 in, 1 out]
            n159 = case shown="\"Debug\"" w433 {
              tunnel: [w438 w440] -> w430
              tunnel: w429 -> [w438 _]
              tunnel: w428 -> [_ w442]
              tunnel: [_ "UI: Front Panel State >> Open\nUI: Wait >> 1000"] -> w423
              frame "Normal", Default {
                # "respect core.close"
              }
              frame "Debug" {
                # "keep panel open\nunless exe"
                n160 = Or(x=w442, y=FALSE) -> (x .or. y?=w440:bool)
              }
            }
            n161 = Bundle By Name(cluster=w426, "Core.Close Panel on Exit?"=w430) -> (w427:T17)
            n162 = call <vilib>:"Add State(s) to Queue__jki_lib_state_machine.vi"("State(s) in Front (\"\")"=w423, "State(s) in (\"\")"=w437) -> ("States Out"=w436:string)  [unwired: 13 in]
          }
          frame "Macro: Transport" {
            # "\"Macro: Transport\" \n()"
            n163 = call <vilib>:"Add State(s) to Queue__jki_lib_state_machine.vi"("State(s) in Front (\"\")"="Transport: prepareTransport\nData: Set Status >> running\nTransport: startTransport\nData: Set Status >> idle" ("State(s) in Front (\"\")"), "State(s) in (\"\")"=w448) -> ("States Out"=w447:string)  [unwired: 13 in]
          }
          frame "Macro: Exit" {
            # "Exit Macro\n(This is called once, when the VI exits)"
            n164 = Unbundle By Name(w450) -> ("Core.Close Panel on Exit?"=w463:bool)
            n165 = Select(t="UI: Front Panel State >> Close", s=w463, f="" ("Empty String Constant")) -> (s? t:f=w461:string)
            n166 = Bundle By Name(cluster=w450, "Core.Shutdown?"=TRUE) -> (w451:T17)
            n167 = call <vilib>:"Add State(s) to Queue__jki_lib_state_machine.vi"("State(s) in Front (\"\")"="Data: Cleanup\nEvents: Unregister\n//Process: Self Terminate", "State(s) in (\"\")"="Process: Sync", "State(s) at Back (\"\")"="Exit") -> ("States Out"=w456:string)  [unwired: 12 in]
            n168 = call <vilib>:"Add State(s) to Queue__jki_lib_state_machine.vi"("State(s) in Front (\"\")"="Sequence: Status >> Shutting down...", "State(s) in (\"\")"=w461, "State(s) at Back (\"\")"=w456) -> ("States Out"=w460:string)  [unwired: 12 in]
            n169 = call <vilib>:"Add State(s) to Queue__jki_lib_state_machine.vi"("State(s) in Front (\"\")"=w460, "State(s) in (\"\")"=w465) -> ("States Out"=w464:string)  [unwired: 13 in]
          }
          frame "---------- Process ----------" {
            # "Template Separator\n(You can make a copy of, or modify, this frame)"
            n170 = call <vilib>:"Add State(s) to Queue__jki_lib_state_machine.vi"("State(s) in (\"\")"=w470) -> ("States Out"=w469:string)  [unwired: 14 in]
          }
          frame "Process: Sync" {
            n171 = Unbundle By Name(w478) -> ("SelfRef"=w474:refnum<class "Inst.Transport.lvclass">)
            n172 = call <vilib>:"WaitOnProcessSync.vi"("error in (no error)"=w473, "SMO"=w474) -> ("error out"=w472:errorcluster, "Don't run?"=w477:bool)  [unwired: 7 in, 1 out]
            n173 = Select(t="Data: Cleanup\nEvents: Unregister\nExit", s=w477, f="" ("Empty String Constant")) -> (s? t:f=w471:string)
            n174 = call <vilib>:"Add State(s) to Queue__jki_lib_state_machine.vi"("State(s) in Front (\"\")"=w471, "State(s) in (\"\")"=w481) -> ("States Out"=w480:string)  [unwired: 13 in]
          }
          frame "Process: Self Terminate" {
            # "Template Separator\n(You can make a copy of, or modify, this frame)"
            n175 = Unbundle By Name(w485) -> ("SelfRef"=w484:refnum<class "Inst.Transport.lvclass">)
            n176 = call <vilib>:"SelfTerminate.vi"("error in (no error)"=w482, "SMO in"=w484) -> ("error out"=w483:errorcluster)  [unwired: 8 in, 1 out]
            n177 = call <vilib>:"Add State(s) to Queue__jki_lib_state_machine.vi"("State(s) in (\"\")"=w488) -> ("States Out"=w487:string)  [unwired: 14 in]
          }
          frame "---------- Events ----------" {
            # "Template Separator\n(You can make a copy of, or modify, this frame)"
            n178 = call <vilib>:"Add State(s) to Queue__jki_lib_state_machine.vi"("State(s) in (\"\")"=w493) -> ("States Out"=w492:string)  [unwired: 14 in]
          }
          frame "Events: Register" {
            n179 = Unbundle By Name(w499) -> ("SelfRef"=w500:refnum<class "Inst.Transport.lvclass">)
            n180 = call <vilib>:"GetProtectedEvents.vi"("SMO"=w500) -> ("error out"=w498:errorcluster, "SMO Protected Events"=w503:T20, "SMO out"=w497:refnum<class "Inst.Transport.lvclass">)  [unwired: 8 in]
            n181 = call "Inst.Transport.GetPrivateEvents.vi"("Inst.Transport in"=w497) -> ("error out"=w494:errorcluster, "Transport Private Events"=w495:cluster{"MessageToProcess":refnum<user-event>})  [unwired: 8 in, 1 out]
            n182 = register-events(w503, w495) -> (reference out=w504:refnum<event-registration>, error out=w501:errorcluster)  [unwired: 2 in]
            n183 = Merge Errors(w501, w494, w498, w496) -> (w502:errorcluster)
            n184 = call <vilib>:"Add State(s) to Queue__jki_lib_state_machine.vi"("State(s) in (\"\")"=w506) -> ("States Out"=w505:string)  [unwired: 14 in]
          }
          frame "Events: Unregister" {
            n185 = Unregister For Events(event registration refnum=w509, error in=w508) -> (error out=w507:errorcluster)
            n186 = call <vilib>:"Clear Errors.vi"("error in (no error)"=w507) -> ()  [unwired: 5 in, 2 out]
            n187 = call <vilib>:"Add State(s) to Queue__jki_lib_state_machine.vi"("State(s) in (\"\")"=w512) -> ("States Out"=w511:string)  [unwired: 14 in]
          }
          frame "---------- Transport ----------" {
            n188 = Unbundle By Name(w515) -> ("SelfRef"=w513:refnum<class "Inst.Transport.lvclass">, "Transport"=w514:refnum<class "Transport.lvclass">)
            n189 = Bundle By Name(cluster=w515, "SelfRef"=w513, "Transport"=w514) -> (w516:T17)
            n190 = call <vilib>:"Add State(s) to Queue__jki_lib_state_machine.vi"("State(s) in (\"\")"=w520) -> ("States Out"=w519:string)  [unwired: 14 in]
          }
          frame "Transport: prepareTransport" {
            n191 = Unbundle By Name(w540) -> ("SelfRef"=w539:refnum<class "Inst.Transport.lvclass">, "Transport"=w522:refnum<class "Transport.lvclass">, "C.E."=w524:refnum<class "Control Experiment.lvclass">, "Comments"=w526:string, "Folder"=w525:string)  [unwired: 1 out]
            n192 = call "Control Experiment FGV.vi"("Function"=enum16{"read", "write"}."read", "error in (no error)"=w530, "Control Experiment.lvclass"=refnum<class "Control Experiment.lvclass"> refnum) -> ("error out"=w535:errorcluster, "Control Experiment.lvclass out"=w537:refnum<class "Control Experiment.lvclass">)  [unwired: 7 in]
            n193 = call "Write Experiment Folder.vi"("error in (no error)"=w535, "Experiment Folder"=w525, "Control Experiment in"=w537) -> ("error out"=w534:errorcluster, "Control Experiment out"=w536:refnum<class "Control Experiment.lvclass">)  [unwired: 7 in]
            n194 = call "Read All Dictionary Elements.vi"("Control Experiment in"=w524) -> ("Items"=w523:T21[])  [unwired: 8 in, 2 out]
            n195 = call "Write Experiment Description.vi"("error in (no error)"=w534, "Experiment Description"=w526, "Control Experiment in"=w536) -> ("error out"=w529:errorcluster, "Control Experiment out"=w533:refnum<class "Control Experiment.lvclass">)  [unwired: 7 in]
            n196 = call "Write Dictionary Elements (Loop).vi"("error in (no error)"=w529, "Data in"=w523, "Control Experiment in"=w533) -> ("error out"=w527:errorcluster, "Control Experiment out"=w532:refnum<class "Control Experiment.lvclass">)  [unwired: 7 in]
            n197 = call "Write Dependencies.vi"("error in (no error)"=w527, "Control Experiment"=w532, "Transport in"=w522) -> ("error out"=w528:errorcluster, "Transport out"=w531:refnum<class "Transport.lvclass">)  [unwired: 7 in]
            n198 = Bundle By Name(cluster=w540, "SelfRef"=w539, "Transport"=w531) -> (w541:T17)
            n199 = call <vilib>:"Add State(s) to Queue__jki_lib_state_machine.vi"("State(s) in (\"\")"=w544) -> ("States Out"=w543:string)  [unwired: 14 in]
          }
          frame "Transport: startTransport" {
            # "notifier is already\non transport\nwire"
            n200 = Unbundle By Name(w553) -> ("Transport"=w551:refnum<class "Transport.lvclass">, "path"=w545:path, "method"=w550:T4, "notifier"=w552:refnum<notifier>)
            n201 = Get Date/Time In Seconds() -> (seconds since 1Jan1904=w546:timestamp)
            n202 = while {
              tunnel: w552 -> [w581]
              tunnel: w551 -> [w589]
              tunnel: w548 -> [w590]
              tunnel: w548 -> [w584]
              tunnel: w545 -> [w588]
              tunnel: w550 -> [w586]
              tunnel: [w577] -> w547
              stop <- w591 stop-if-true
              # "repeat until stop notifier is received"
              n203 = call "Inst.Transport.CallByReference.vi"("error in (no error)"=w590, "VI"=w586, "vi path"=w588, "Transport"=w589) -> ("error out"=w585:errorcluster)  [unwired: 7 in]
              n204 = Merge Errors(w585, w584) -> (w577:errorcluster)
              n205 = Equal?(x=Inst.Transport.Methods--Enum."LockinTimeDelay" ("input 1"), y=w586) -> (x = y?=w583:bool)
              n206 = Get Notifier Status(notifier=w581, error in (no error)=w577) -> (notifier out=w582:refnum<notifier>, current notification=w580:bool, error out=w579:errorcluster)  [unwired: 2 out]
              n207 = Send Notification(notification=w583, notifier=w582) -> (error out=w578:errorcluster)  [unwired: 1 in, 1 out]
              n208 = Compound Arithmetic op=OR(w578, w583, w580, w579) -> (w591:bool)
            }
            n209 = while {
              tunnel: w552 -> [w570]
              tunnel: w548 -> [_]
              tunnel: w546 -> [w562]
              stop <- w565 stop-if-true
              n210 = Get Date/Time In Seconds() -> (seconds since 1Jan1904=w563:timestamp)
              n211 = Subtract(x=w563, y=w562) -> (x-y=w557:dbl)
              n212 = local read "Secret Status"() -> (w559:string)
              n213 = case shown="False" "stopTransport" {
                selector: "stopTransport" -> [_ w573]
                tunnel: w570 -> [w571 w576]
                tunnel: [w571 w575] -> w569
                tunnel: [_ w574] -> w568
                frame False {
                }
                frame True {
                  n214 = local write "stopTransport"(FALSE ("stopTransport")) -> ()
                  n215 = Send Notification(notification=w573, notifier=w576) -> (notifier out=w575:refnum<notifier>, error out=w574:errorcluster)  [unwired: 1 in]
                }
              }
              n216 = Format Into String(format string=" %.3f s", initial string=w559, w557) -> (resulting string=w558:string)  [unwired: 1 in, 1 out]
              n217 = local write "Status"(w558) -> ()
              n218 = Get Notifier Status(notifier=w569, error in (no error)=w568) -> (current notification=w566:bool, error out=w567:errorcluster)  [unwired: 3 out]
              n219 = Or(x=w566, y=w567) -> (x .or. y?=w565:bool)
              n220 = Wait (ms)(milliseconds to wait=u32 100) -> ()  [unwired: 1 out]
            }
            n221 = Merge Errors(w547, w548) -> (w549:errorcluster)
            n222 = call <vilib>:"Add State(s) to Queue__jki_lib_state_machine.vi"("State(s) in (\"\")"=w556) -> ("States Out"=w555:string)  [unwired: 14 in]
          }
          frame "Transport: appendExptParam" {
            n223 = Unbundle By Name(w600) -> ("C.E."=w599:refnum<class "Control Experiment.lvclass">, "MessageToProcess.Message.Data"=w592:variant)
            n224 = call "Parse ExptParam.vi"("error in (no error)"=w594, "params in"=w592) -> ("error out"=w593:errorcluster, "value"=w595:variant, "key"=w596:string)  [unwired: 7 in]
            n225 = call "Append Dictionary Element.vi"("error in (no error)"=w593, "value"=w595, "key"=w596, "Control Experiment in"=w599) -> ("error out"=w597:errorcluster, "Control Experiment out"=w598:refnum<class "Control Experiment.lvclass">)  [unwired: 6 in]
            n226 = Bundle By Name(cluster=w600, "C.E."=w598) -> (w601:T17)
            n227 = call <vilib>:"Add State(s) to Queue__jki_lib_state_machine.vi"("State(s) in (\"\")"=w604) -> ("States Out"=w603:string)  [unwired: 14 in]
          }
          frame "Transport: setExptParam" {
            n228 = Unbundle By Name(w613) -> ("C.E."=w612:refnum<class "Control Experiment.lvclass">, "MessageToProcess.Message.Data"=w609:variant)
            n229 = call "Parse ExptParam.vi"("error in (no error)"=w608, "params in"=w609) -> ("error out"=w607:errorcluster, "value"=w605:variant, "key"=w606:string)  [unwired: 7 in]
            n230 = call "Write Dictionary Element.vi"("error in (no error)"=w607, "value"=w605, "key"=w606, "Control Experiment in"=w612) -> ("error out"=w610:errorcluster, "Control Experiment out"=w611:refnum<class "Control Experiment.lvclass">)  [unwired: 6 in]
            n231 = Bundle By Name(cluster=w613, "C.E."=w611) -> (w614:T17)
            n232 = call <vilib>:"Add State(s) to Queue__jki_lib_state_machine.vi"("State(s) in (\"\")"=w617) -> ("States Out"=w616:string)  [unwired: 14 in]
          }
          frame "Transport: clearExptParam" {
            n233 = Bundle By Name(cluster=w619, "C.E."=refnum<class "Control Experiment.lvclass"> refnum) -> (w620:T17)
            n234 = call <vilib>:"Add State(s) to Queue__jki_lib_state_machine.vi"("State(s) in (\"\")"=w624) -> ("States Out"=w623:string)  [unwired: 14 in]
          }
          frame "Transport: setSweepConfig" {
            n235 = Unbundle By Name(w639) -> ("Transport"=w637:refnum<class "Transport.lvclass">, "MessageToProcess.Message.Data"=w636:variant)
            n236 = call "JSON to LVtype.vim"("type"=T10 {"sweepTime"=0.0, "initialWaitTime"=0.0, "returnToStart"=FALSE, "sweepChannels"=[{"Enable?"=FALSE, "Channel"=0, "Start"=0.0, "End"=0.1, "Pattern"=enum."Ramp /", "Table"=[1.0]}]} ("setSweepConfig"), "error in (no error)"=w634, "JSON Data in"=w636) -> ("error out"=w635:errorcluster, "Data out"=w626:T10)  [unwired: 7 in]
            n237 = Unbundle By Name(w626) -> ("sweepTime"=w631:dbl, "initialWaitTime"=w630:dbl, "returnToStart"=w629:bool, "sweepChannels"=w628:T11)
            n238 = Bundle By Name(cluster=T14 {"Sweep Time (s)"=0.0, "Initial Wait (s)"=0.0, "Return to Start"=FALSE, "Sweep Channels"=[], "Sweep Tables"=[]} ("Lockin_Sweep"), "Sweep Time (s)"=w631, "Initial Wait (s)"=w630, "Return to Start"=w629, "Sweep Channels"=w628) -> (w625:T14)
            n239 = call "Write Configure Sweep.vi"("error in (no error)"=w635, "Lockin_Sweep"=w625, "Transport in"=w637) -> ("error out"=w633:errorcluster, "Transport out"=w638:refnum<class "Transport.lvclass">)  [unwired: 7 in]
            n240 = Bundle By Name(cluster=w639, "Transport"=w638) -> (w640:T17)
            n241 = call <vilib>:"Add State(s) to Queue__jki_lib_state_machine.vi"("State(s) in (\"\")"=w643) -> ("States Out"=w642:string)  [unwired: 14 in]
          }
          frame "Transport: Log" {
            # "THIS process.vi is responsible for logging data. Logging can be triggered in the timeout (as shown in this template proces.vi's tieout case) OR it could be triggered by data changes, or any other way you can device.\n\nThe code above will log ALL data. But you have the ability to log a subset, log some items on a different schedule, etc."
            n242 = Unbundle By Name(w652) -> ("SelfRef"=w648:refnum<class "Inst.Transport.lvclass">)
            n243 = call-dynamic "Get SMO Database Paths.vi"("error in (no error)"=w645, "Inst.Transport in"=w648) -> ("error out"=w646:errorcluster, "Paths"=w649:string, "Inst.Transport out"=w644:refnum<class "Inst.Transport.lvclass">)  [unwired: 7 in]
            n244 = Unbundle By Name(w644) -> ("Data"=w647:T22)
            n245 = call <userlib>:"Instrument.logToDatabase.vi"("error in (no error)"=w646, "Data"=w647, "Paths"=w649, "Instrument"=w644) -> ("error out"=w650:errorcluster, "Instrument out"=w651:refnum<class "Inst.Transport.lvclass">)  [unwired: 6 in]
            n246 = Bundle By Name(cluster=w652, "SelfRef"=w651) -> (w653:T17)
            n247 = call <vilib>:"Add State(s) to Queue__jki_lib_state_machine.vi"("State(s) in (\"\")"=w656) -> ("States Out"=w655:string)  [unwired: 14 in]
          }
          frame "---------- Sequence ----------" {
            n248 = call <vilib>:"Add State(s) to Queue__jki_lib_state_machine.vi"("State(s) in (\"\")"=w661) -> ("States Out"=w660:string)  [unwired: 14 in]
          }
          frame "Sequence: Status" {
            # "Sequence: Status\n(Use this frame to pass the status to the UI, this VI's UI, etc)"
            n249 = call <vilib>:"Add State(s) to Queue__jki_lib_state_machine.vi"("State(s) in (\"\")"=w667) -> ("States Out"=w666:string)  [unwired: 14 in]
            "Secret Status" <- w662
            "Status" <- w662
          }
          frame "Sequence: Wait" {
            # "Sequence: Wait\n(Non-Blocking Wait)"
            # "F = repeat this state. wait\nT = go to next state. don't wait"
            n250 = Unbundle By Name(w676) -> ("Running Step"=w669:i32)
            n251 = call <userlib>:"Wait Logic.vi"("error in (no error)"=w672, "Time"=w670) -> ("error out"=w671:errorcluster, "Status String"=w668:string, "Trigger"=w673:bool)  [unwired: 6 in, 1 out]
            n252 = Increment(x=w669) -> (x+1=w683:i32)
            n253 = Select(t=w683, s=w673, f=w669) -> (s? t:f=w674:i32)
            n254 = Select(t=u32 0, s=w673, f=u32 100 ("milliseconds to wait")) -> (s? t:f=w680:u32)
            n255 = call <userlib>:"Wait (ms)__ogtk.vi"("error in (no error)"=w671, "milliseconds to wait"=w680) -> ("error out"=w678:errorcluster)  [unwired: 8 in, 1 out]
            n256 = Bundle By Name(cluster=w676, "Running Step"=w674) -> (w675:T17)
            n257 = call <vilib>:"Build State String with Arguments__JKI_lib_State_Machine.vi"("Arguments (\"\")"=w668, "State"="Sequence: Status") -> ("State with Arguments"=w677:string)  [unwired: 4 in]
            n258 = call <vilib>:"Add State(s) to Queue__jki_lib_state_machine.vi"("State(s) in Front (\"\")"=w677, "State(s) in (\"\")"=w686) -> ("States Out"=w685:string)  [unwired: 13 in]
          }
        }
      }
    }
    frame Error {
    }
  }
  n259 = call-parent "Process.vi"("error in"=w3, "Instrument"=w6) -> ("error out"=w5:errorcluster, "Instrument out"=→"Inst.Transport out":refnum<class "Inst.Transport.lvclass">)  [unwired: 8 in]
  n260 = Merge Errors(w5, w4) -> (→"error out":errorcluster)
